vi "Read Discrete Inputs.vi"(8 "error in (no error)":errorcluster, 9 "number of discrete inputs":u16, 10 "starting address":u16, 11 "Modbus master in":refnum<class "Network Master.lvclass">) -> (0 "error out":errorcluster, 2 "discrete input values":bool[](array[boolean]), 3 "Modbus master out":refnum<class "Network Master.lvclass">)   [LabVIEW 2021, in "Network Master.lvclass"]
doc: "Reads values from contiguous discrete inputs. The maximum number of discrete inputs this VI can read is 2,000."
uses:
  Network Master.lvclass
  D:/my_projects/projects/Algorithms/Labview/21/Modbus_v121c/Network Protocol/Network Protocol.lvclass
  Modbus Data Unit/Modbus Data Unit.lvclass/Modbus Data Unit.ctl
  Network Protocol.lvclass/Network Protocol.ctl
  Network Master.lvclass/Network Master.ctl
  Modbus Data Unit/Construct PDU.vi
  Read Transmission Data Unit.vi
  Utility/Bytes to Bits.vi
  Master Function Definition/Function code mismatch error.vi
  Data Model/Error Generator.vi
  Modbus Data Unit/Deconstruct PDU.vi
  Modbus Data Unit/Modbus Data Unit.lvclass
  Transmission Data Unit/Transmission Data Unit.lvclass
  Master Function Definition/Master Function Definition.lvclass
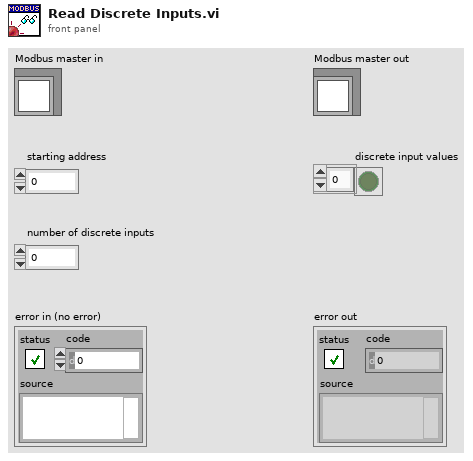
[diagram p1: front panel]
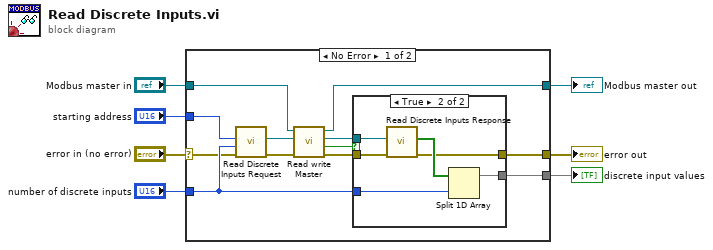
[diagram p0: block diagram]
diagram:
  n1 = case shown="No Error" "error in (no error)" {
    selector: "error in (no error)" -> [w10 w27]
    tunnel: "Modbus master in" -> [w8 w28]
    tunnel: [w9 w28] -> w6
    tunnel: [w14 w27] -> w5
    tunnel: [w17 _] -> w3
    tunnel: "number of discrete inputs" -> [w16 _]
    tunnel: "starting address" -> [w18 _]
    frame No Error {
      n2 = call "Read Discrete Inputs Request.vi"("error in"=w10, "Number of inputs"=w16, "starting address"=w18) -> ("error out"=w19:errorcluster, "modbus data unit out"=w11:refnum<class "Modbus Data Unit.lvclass">)  [unwired: 7 in]
      n3 = call "Read write Master.vi"("error in (no error)"=w19, "Modbus data unit in"=w11, "Modbus master in"=w8) -> ("error out"=w15:errorcluster, "PDU valid?"=w13:bool, "Modbus data unit out"=w12:refnum<class "Modbus Data Unit.lvclass">, "Modbus master out"=w9:refnum<class "Network Master.lvclass">)  [unwired: 5 in]
      n4 = case shown="True" w13 {
        tunnel: [_ w25] -> w17
        tunnel: w16 -> [_ w24]
        tunnel: w15 -> [w20 w23]
        tunnel: w12 -> [_ w22]
        tunnel: [w20 w21] -> w14
        frame False {
        }
        frame True {
          n5 = call "Read Discrete Inputs Response.vi"("error in"=w23, "modbus data unit in"=w22) -> ("error out"=w21:errorcluster, "Data"=w26:bool[])  [unwired: 8 in]
          n6 = Split 1D Array(array=w26, index=w24) -> (first subarray=w25:bool[])  [unwired: 1 out]
        }
      }
    }
    frame Error {
    }
  }
  "error out" <- w5
  "Modbus master out" <- w6
  "discrete input values" <- w3
